vi "FeedbackDecode_20200902.vi"() -> ()   [LabVIEW 2016] (continued)
  out "prevWAVChart":dbl[](graph)=[0.01885986328125, 0.02471923828125, 0.026458740234375, 0.019622802734375, 0.015625, 0.016571044921875, 0.017852783203125, 0.016937255859375, 0.02349853515625, 0.0262451171875, 0.021697998046875, 0.01995849609375, 0.013427734375, 0.008819580078125, 0.013916015625, 0.016693115234375, 0.0172119140625, 0.023468017578125, 0.0235595703125, 0.018890380859375, 0.022369384765625, 0.022003173828125, 0.019378662109375, 0.017578125, 0.0115966796875, 0.011688232421875, 0.011016845703125, 0.007659912109375, 0.012359619140625, 0.015167236328125, 0.010162353515625, 0.00787353515625, 0.010009765625, 0.01434326171875, 0.018524169921875, 0.019012451171875, 0.019317626953125, 0.019500732421875, 0.021514892578125, 0.021514892578125, 0.0233154296875, 0.02276611328125, 0.0174560546875, 0.018585205078125, 0.019439697265625, 0.01959228515625, 0.0185546875, 0.015594482421875, 0.01593017578125, 0.0162353515625, 0.013427734375, 0.01519775390625, 0.005340576171875, 0.008026123046875, 0.00811767578125, 0.004669189453125, 0.008148193359375, 0.00384521484375, 0.007598876953125, 0.007354736328125, 0.009735107421875, 0.01580810546875, 0.01385498046875, 0.014923095703125, 0.00830078125, 0.005096435546875, 0.008941650390625, 0.01416015625, 0.01220703125, 0.0140380859375, 0.01275634765625, 0.006439208984375, 0.007049560546875, 0.006134033203125, -0.000457763671875, 0.003326416015625, 0.0081787109375, 0.009124755859375, 0.013458251953125, 0.014007568359375, 0.014312744140625, 0.006011962890625, 0.00238037109375, 0.010284423828125, 0.011962890625, 0.009857177734375, 0.00909423828125, 0.016448974609375, 0.01885986328125, 0.01190185546875, 0.010955810546875, 0.01019287109375, 0.00152587890625, 0.00762939453125, 0.008270263671875, 0.00604248046875, 0.010589599609375, 0.0037841796875, 0.0050048828125, 0.007080078125, 0.004669189453125, 0.0064697265625, 0.01068115234375, 0.009521484375, 0.002532958984375, -0.000518798828125, 0.005035400390625, 0.0042724609375, 0.00164794921875, 0.0001220703125, -0.002716064453125, -0.00164794921875, -0.007232666015625, -0.01153564453125, -0.005889892578125, -0.00341796875, -0.008514404296875, -0.007415771484375, -0.00726318359375, -0.007781982421875, -0.009918212890625, -0.010772705078125, -0.00628662109375, -0.001373291015625, -0.0008544921875, -0.003997802734375, 0.003021240234375, 0.003082275390625, 0.000640869140625, 0.00250244140625, 0.002960205078125, 0.00115966796875, 0.000579833984375, -0.002166748046875, -0.00115966796875, -0.006591796875, -0.0128173828125, -0.013275146484375, -0.0157470703125, -0.016204833984375, -0.013885498046875, -0.01531982421875, -0.00897216796875, -0.00762939453125, -0.00738525390625, -0.00311279296875, -0.002166748046875, 0.000244140625, -0.003509521484375, -0.003662109375, 0.001220703125, 0.001251220703125, 0.0001220703125, -0.003692626953125, -0.003997802734375, -0.004364013671875, -9.1552734375e-05, 0.00341796875, 0.000457763671875, -0.000274658203125, -0.0006103515625, 0.00543212890625, 0.001312255859375, 0.003662109375, 0.009765625, 0.004852294921875, 0.003997802734375, 0.00189208984375, -0.000213623046875, -0.006500244140625, -0.006744384765625, -0.0120849609375, -0.012359619140625, -0.003631591796875, -0.005645751953125, -0.0028076171875, 0.00286865234375, -0.00311279296875, -0.005279541015625, 0.001922607421875, -0.003753662109375, -0.000335693359375, -0.00299072265625, 0.001556396484375, 0.00299072265625, 0.006317138671875, 0.006622314453125, -0.003692626953125, -0.007110595703125, 0.001190185546875, -0.002288818359375, 0.00030517578125, 0.007720947265625, 0.003692626953125, 0.006011962890625, 0.007904052734375, 0.0115966796875, 0.01513671875, 0.00421142578125, 0.00299072265625, 0.002532958984375, 0.0009765625, 0.0018310546875, 0.001556396484375, 0.00640869140625, 0.008148193359375, 0.011962890625, 0.01416015625, 0.01055908203125, 0.0126953125, 0.006500244140625, 0.00958251953125, 0.009613037109375, 0.00921630859375, 0.007049560546875, 0.00927734375, 0.011871337890625, 0.015655517578125, 0.0146484375, 0.011627197265625, 0.0162353515625, 0.007965087890625, 0.00146484375, 0.004425048828125, 0.007415771484375, 0.007598876953125, 0.011810302734375, 0.01324462890625, 0.016357421875, 0.0126953125, 0.012451171875, 0.01763916015625, 0.0196533203125, 0.019775390625, 0.021453857421875, 0.025848388671875, 0.023468017578125, 0.01934814453125, 0.019073486328125, 0.020355224609375, 0.021270751953125, 0.024139404296875, 0.02545166015625, 0.0255126953125, 0.027862548828125, 0.027435302734375, 0.030487060546875, 0.029052734375, 0.032196044921875, 0.030120849609375, 0.035552978515625, 0.026611328125, 0.025787353515625, 0.030303955078125, 0.021270751953125, 0.027099609375, 0.032379150390625, 0.03143310546875, 0.02508544921875, 0.03118896484375, 0.029510498046875, 0.0311279296875, 0.03460693359375, 0.0340576171875, 0.027435302734375, 0.03076171875, 0.031707763671875, 0.029815673828125, 0.0341796875, 0.039337158203125, 0.0396728515625, 0.039459228515625, 0.031463623046875, 0.025482177734375, 0.03057861328125, 0.031707763671875, 0.03253173828125, 0.035308837890625, 0.0355224609375, 0.035369873046875, 0.02996826171875, 0.0267333984375, 0.025665283203125, 0.024688720703125, 0.029754638671875, 0.023681640625, 0.02490234375, 0.026458740234375, 0.025726318359375, 0.03436279296875, 0.028411865234375, 0.0225830078125, 0.02349853515625, 0.021270751953125, 0.02691650390625, 0.02520751953125, 0.023101806640625, 0.020782470703125, 0.0198974609375, 0.024200439453125, 0.021148681640625, 0.023406982421875, 0.028289794921875, 0.02862548828125, 0.03240966796875, 0.025634765625, 0.030120849609375, 0.029998779296875, 0.02752685546875, 0.033660888671875, 0.028167724609375, 0.032073974609375, 0.033233642578125, 0.02862548828125, 0.029876708984375, 0.02667236328125, 0.02392578125, 0.02764892578125, 0.026275634765625, 0.023468017578125, 0.031158447265625, 0.0306396484375, 0.022125244140625, 0.022430419921875, 0.025054931640625, 0.02337646484375, 0.025299072265625, 0.02777099609375, 0.03326416015625, 0.02777099609375, 0.025390625, 0.028778076171875, 0.02239990234375, 0.01837158203125, 0.021148681640625, 0.021514892578125, 0.018218994140625, 0.01593017578125, 0.017547607421875, 0.018524169921875, 0.01739501953125, 0.01922607421875, 0.016632080078125, 0.010772705078125, 0.013519287109375, 0.011383056640625, 0.013671875, 0.017242431640625, 0.021636962890625, 0.01922607421875, 0.01593017578125, 0.016571044921875, 0.015777587890625, 0.016693115234375, 0.011260986328125, 0.005828857421875, 0.0068359375, 0.001739501953125, 0.00518798828125, 0.006591796875, 0.00286865234375, 0.015289306640625, 0.011383056640625, 0.01031494140625, 0.00927734375, 0.009307861328125, 0.011199951171875, 0.010894775390625, 0.006927490234375, 0.0115966796875, 0.004638671875, 0.004425048828125, 0.003631591796875, 0.007659912109375, 0.0086669921875, 0.00616455078125, 0.003509521484375, -0.000518798828125, 0.0001220703125, -0.001708984375, -0.0015869140625, 0.002349853515625, 0.0089111328125, 0.007171630859375, 0.0072021484375, 0.004791259765625, 0.00341796875, 0.001068115234375, 0.00341796875, 0.00445556640625, 0.008056640625, 0.009246826171875, 0.011077880859375, 0.006195068359375, 0.005340576171875, 0.00244140625, 0.006561279296875, 0.016021728515625, 0.011322021484375, 0.0079345703125, 0.006622314453125, 0.01080322265625, 0.009796142578125, 0.0028076171875, 0.00439453125, 0.00048828125, 0.0052490234375, 0.0025634765625, 0.00396728515625, 0.0057373046875, 0.00860595703125, 0.00701904296875, 0.0020751953125, -0.00189208984375, -0.001861572265625, 0.00091552734375, -0.00762939453125, -0.0074462890625, -0.0054931640625, 0.0010986328125, 0.00421142578125, 0.001800537109375, 0.007232666015625, -0.001190185546875, 9.1552734375e-05, -0.0078125, -0.010833740234375, -0.0068359375, -0.0054931640625, -0.004791259765625, -0.011016845703125, -0.009765625, -0.007720947265625, -0.00384521484375, -0.011260986328125, -0.00848388671875, -0.000152587890625, -0.00030517578125, -0.00177001953125, -0.0052490234375, -0.00994873046875, -0.001617431640625, -0.00567626953125, -0.008209228515625, -0.004638671875, -0.0057373046875, -0.0067138671875, -0.01080322265625, -0.008544921875, -0.0120849609375, -0.009857177734375, -0.01409912109375, -0.0184326171875, -0.022003173828125, -0.023101806640625, -0.02197265625, -0.021942138671875, -0.018035888671875, -0.016632080078125, -0.025726318359375, -0.032623291015625, -0.02557373046875, -0.03179931640625, -0.020660400390625, -0.017578125, -0.01641845703125, -0.017852783203125, -0.02423095703125, -0.030609130859375, -0.03009033203125, -0.027862548828125, -0.031646728515625, -0.03076171875, -0.0225830078125, -0.015472412109375, -0.018341064453125, -0.02520751953125, -0.032958984375, -0.034759521484375, -0.034637451171875, -0.033233642578125, -0.031768798828125, -0.025238037109375, -0.02752685546875, -0.03057861328125, -0.0286865234375, -0.03204345703125, -0.02850341796875, -0.020965576171875, -0.022735595703125, -0.02435302734375, -0.024383544921875, -0.02496337890625, -0.01910400390625, -0.0230712890625, -0.0225830078125, -0.02435302734375, -0.027984619140625, -0.027740478515625, -0.026153564453125, -0.03021240234375, -0.030792236328125, -0.0277099609375, -0.0250244140625, -0.02239990234375, -0.025146484375, -0.029571533203125, -0.022491455078125, -0.02587890625, -0.02081298828125, -0.024688720703125, -0.026885986328125, -0.026214599609375, -0.025482177734375, -0.027374267578125, -0.03387451171875, -0.03570556640625, -0.0379638671875, -0.03662109375, -0.034637451171875, -0.03826904296875, -0.0408935546875, -0.037384033203125, -0.038177490234375, -0.039337158203125, -0.03564453125, -0.02972412109375, -0.02410888671875, -0.01873779296875, -0.02288818359375, -0.02679443359375, -0.03839111328125, -0.0316162109375, -0.029449462890625, -0.02972412109375, -0.03564453125, -0.034332275390625, -0.038665771484375, -0.044525146484375, -0.040374755859375, -0.039031982421875, -0.03741455078125, -0.039703369140625, -0.0386962890625, -0.036834716796875, -0.03521728515625, -0.033905029296875, -0.02984619140625, -0.035430908203125, -0.032440185546875, -0.029022216796875, -0.024688720703125, -0.024139404296875, -0.027099609375, -0.027313232421875, -0.02496337890625, -0.02203369140625, -0.0244140625, -0.021240234375, -0.02392578125, -0.020782470703125, -0.01873779296875, -0.0208740234375, -0.0208740234375, -0.022491455078125, -0.01806640625, -0.0216064453125, -0.017181396484375, -0.01397705078125, -0.01556396484375, -0.009979248046875, -0.016693115234375, -0.01068115234375, -0.016754150390625, -0.01959228515625, -0.016143798828125, -0.02447509765625, -0.029266357421875, -0.026947021484375, -0.02496337890625, -0.0345458984375, -0.027618408203125, -0.0318603515625, -0.028656005859375, -0.02685546875, -0.025634765625, -0.02392578125, -0.026031494140625, -0.014617919921875, -0.018585205078125, -0.021697998046875, -0.019317626953125, -0.02044677734375, -0.0184326171875, -0.018951416015625, -0.022125244140625, -0.019073486328125, -0.02203369140625, -0.0224609375, -0.02166748046875, -0.019073486328125, -0.015411376953125, -0.016448974609375, -0.023834228515625, -0.021728515625, -0.016387939453125, -0.009490966796875, -0.012542724609375, -0.0169677734375, -0.017822265625, -0.02105712890625, -0.017913818359375, -0.016815185546875, -0.01983642578125, -0.0179443359375, -0.0123291015625, -0.01129150390625, -0.01324462890625, -0.015869140625, -0.01385498046875, -0.016387939453125, -0.015655517578125, -0.0181884765625, -0.017578125, -0.013092041015625, -0.008331298828125, -0.007781982421875, -0.00439453125, -0.007080078125, -0.010223388671875, -0.01239013671875, -0.014923095703125, -0.01080322265625, -0.001983642578125, -0.0074462890625, -0.017791748046875, -0.023040771484375, -0.02978515625, -0.0267333984375, -0.0224609375, -0.017120361328125, -0.024871826171875, -0.01788330078125, -0.012298583984375, -0.011566162109375, -0.00726318359375, -0.00457763671875, -0.00299072265625, 0.00146484375, -0.0037841796875, -0.008819580078125, -0.0076904296875, -0.006256103515625, 0.001373291015625, -0.001708984375, -0.00335693359375, 0.001953125, 0.005859375, 0.00396728515625, 0.007110595703125, 0.011993408203125, 0.005828857421875, 0.00677490234375, 0.000244140625, 0.008575439453125, 0.0098876953125, 0.003875732421875, 0.0067138671875, 0.000946044921875, 0.00274658203125, 0.001800537109375, 0.00506591796875, 0.006072998046875, -0.006103515625, -0.00909423828125, -0.003936767578125, -0.001861572265625, -0.002777099609375, 0.001495361328125, 0.0006103515625, -0.003265380859375, -0.0003662109375, 0.00128173828125, 0.0010986328125, 0.002655029296875, -0.005615234375, -0.01275634765625, -0.00775146484375, -0.004913330078125, -0.004119873046875, -0.00506591796875, -9.1552734375e-05, 0.003204345703125, -0.002410888671875, -0.001800537109375, 0.001312255859375, 0.003173828125, -0.002899169921875, -0.004608154296875, 0.002593994140625, -0.002685546875, -0.00762939453125, -0.0028076171875, -0.006805419921875, -0.0146484375, -0.009979248046875, -0.00177001953125, 0.00286865234375, -0.0091552734375, -0.01495361328125, -0.01080322265625, -0.009368896484375, 0.0023193359375, -0.0010986328125, -0.001678466796875, -0.00177001953125, -0.006134033203125, -0.004730224609375, -0.00921630859375, -0.00909423828125, -0.0108642578125, -0.017181396484375, -0.015289306640625, -0.01458740234375, -0.013336181640625, -0.0057373046875, -0.004852294921875, -0.005645751953125, -0.0050048828125, -0.006500244140625, -0.00927734375, -0.012908935546875, -0.014404296875, -0.0155029296875, -0.0115966796875, -0.009796142578125, -0.01202392578125, -0.018157958984375, -0.021240234375, -0.015533447265625, -0.01629638671875, -0.01318359375, -0.015594482421875, -0.020721435546875, -0.017974853515625, -0.02056884765625, -0.02264404296875, -0.01654052734375, -0.01702880859375, -0.0146484375, -0.013275146484375, -0.023040771484375, -0.015960693359375, -0.013092041015625, -0.011077880859375, -0.009063720703125, -0.01727294921875, -0.018035888671875, -0.01580810546875, -0.011932373046875, -0.01287841796875, -0.003692626953125, -0.015167236328125, -0.014068603515625, -0.01666259765625, -0.0211181640625, -0.01812744140625, -0.013336181640625, -0.01519775390625, -0.0093994140625, -0.012847900390625, -0.0208740234375, -0.01300048828125, -0.006988525390625, -0.006072998046875, -0.011199951171875, -0.01263427734375, -0.01263427734375, -0.015625, -0.01055908203125, -0.00372314453125, -0.001312255859375, 0.001861572265625, -6.103515625e-05, -0.00311279296875, -0.001251220703125, -0.006500244140625, -0.00665283203125, 0.000823974609375, 0.001190185546875, 0.004486083984375, -0.004638671875, -0.00250244140625, -0.000518798828125, 0.001739501953125, 0.010955810546875, 0.00384521484375, -0.002349853515625, -0.00128173828125, -0.002227783203125, -0.005157470703125, -0.003204345703125, -0.00482177734375, -0.006072998046875, -0.001312255859375, -0.00018310546875, 0.0001220703125, -0.000274658203125, 0.003753662109375, 0.0103759765625, 0.009063720703125, 0.01324462890625, 0.019989013671875, 0.01324462890625, 0.015350341796875, 0.017791748046875, 0.019744873046875, 0.0157470703125, 0.007049560546875, 0.01263427734375, 0.0111083984375, 0.009002685546875, 0.01141357421875, 0.016632080078125, 0.012847900390625, 0.007568359375, 0.0042724609375, -0.00372314453125, -0.011383056640625, 0.00128173828125, 0.014312744140625, 0.016082763671875, 0.021697998046875, 0.020172119140625, 0.021575927734375, 0.02032470703125, 0.02215576171875, 0.02471923828125, 0.0302734375, 0.02752685546875, 0.02667236328125, 0.026580810546875, 0.0250244140625, 0.027557373046875, 0.020172119140625, 0.0247802734375, 0.02978515625, 0.030120849609375, 0.03131103515625, 0.031524658203125, 0.032257080078125, 0.0286865234375, 0.03033447265625, 0.0279541015625, 0.03582763671875, 0.036285400390625, 0.03515625, 0.028656005859375, 0.0311279296875, 0.033599853515625, 0.03582763671875, 0.028839111328125, 0.02947998046875, 0.0306396484375, 0.025146484375, 0.020843505859375, 0.027679443359375, 0.028045654296875, 0.02532958984375, 0.024017333984375, 0.02410888671875, 0.032073974609375, 0.018951416015625, 0.02801513671875, 0.0318603515625, 0.02587890625, 0.02825927734375, 0.025421142578125, 0.033203125, 0.03515625, 0.0362548828125, 0.030975341796875, 0.034332275390625, 0.02392578125, 0.027191162109375, 0.03472900390625, 0.03515625, 0.02813720703125, 0.0291748046875, 0.028717041015625, 0.027099609375, 0.02874755859375, 0.02203369140625, 0.019805908203125, 0.0179443359375, 0.0289306640625, 0.023773193359375, 0.017059326171875, 0.020904541015625, 0.0262451171875, 0.022979736328125, 0.021453857421875, 0.024017333984375, 0.02056884765625, 0.022430419921875, 0.02081298828125, 0.021759033203125, 0.026611328125, 0.033660888671875, 0.027374267578125, 0.02435302734375, 0.0185546875, 0.018096923828125, 0.023223876953125, 0.01654052734375, 0.015899658203125, 0.009490966796875, 0.00897216796875, 0.00933837890625, 0.013763427734375, 0.01470947265625, 0.021392822265625, 0.0238037109375, 0.022979736328125, 0.025665283203125, 0.0169677734375, 0.0174560546875, 0.015472412109375, 0.012786865234375, 0.011688232421875, 0.0103759765625, 0.00640869140625, 0.0113525390625, 0.0142822265625, 0.012603759765625, 0.0142822265625, 0.016815185546875, 0.020782470703125, 0.012237548828125, 0.008392333984375, 0.017578125, 0.019775390625, 0.026336669921875, 0.02557373046875, 0.019317626953125, 0.015380859375, 0.0196533203125, 0.01812744140625, 0.020050048828125, 0.015045166015625, 0.01416015625, 0.01129150390625, 0.00885009765625, 0.00799560546875, 0.01055908203125, 0.0107421875, 0.0164794921875, 0.0133056640625, 0.0064697265625, 0.0089111328125, 0.0069580078125, 0.0064697265625, 0.001220703125, -0.003082275390625, -0.0028076171875, -9.1552734375e-05, 0.00201416015625, -0.000946044921875, -0.001495361328125, 0.000579833984375, 0.003265380859375, 0.00390625, 0.005889892578125, 0.002685546875, -0.000732421875, 0.004058837890625, 0.0023193359375, 0.008544921875, 0.00250244140625, -0.000885009765625, -0.00244140625, -0.004608154296875, -0.002288818359375, -0.0050048828125, -0.000885009765625, -0.0013427734375, 0.001800537109375, 0.001678466796875, -0.005279541015625, 0.00506591796875, 0.002899169921875, 0.003662109375, 0.0087890625, 0.011474609375, 0.01422119140625, 0.01055908203125, 0.011444091796875, 0.012359619140625, 0.001190185546875, 0.0054931640625, 0.007598876953125, 0.01025390625, 0.01300048828125, 0.008575439453125, 0.007659912109375, 0.00897216796875, 0.014892578125, 0.01226806640625, 0.014434814453125, 0.022003173828125, 0.02056884765625, 0.022705078125, 0.02532958984375, 0.02154541015625, 0.02130126953125, 0.01788330078125, 0.016845703125, 0.018524169921875, 0.015167236328125, 0.01947021484375, 0.017578125, 0.01470947265625, 0.015533447265625, 0.015594482421875, 0.00836181640625, 0.0164794921875, 0.017608642578125, 0.012481689453125, 0.01287841796875, 0.01123046875, 0.010986328125, 0.01324462890625, 0.015655517578125, 0.01287841796875, 0.0107421875, 0.012908935546875, 0.00885009765625, 0.00201416015625, 0.008026123046875, 0.00994873046875, 0.011444091796875, 0.010894775390625, 0.01385498046875, 0.0174560546875, 0.014495849609375, 0.009246826171875, 0.00982666015625, 0.010406494140625, 0.015411376953125, 0.01507568359375, 0.0067138671875, 0.009521484375, 0.011322021484375, 0.00811767578125, -0.002410888671875, 0.00299072265625, -0.004852294921875, 0.0032958984375, 0.0032958984375, 6.103515625e-05, 0.00152587890625, 0.003082275390625, 0.011627197265625, 0.013458251953125, 0.01239013671875, 0.015777587890625, 0.023406982421875, 0.027923583984375, 0.024139404296875, 0.020721435546875, 0.022308349609375, 0.026519775390625, 0.019256591796875, 0.013214111328125, 0.0146484375, 0.015777587890625, 0.02001953125, 0.0150146484375, 0.01055908203125, 0.00897216796875, 0.00823974609375, 0.0013427734375, 0.005615234375, -0.00225830078125, -0.008087158203125, 0.005950927734375, 0.00762939453125, 0.003326416015625, 0.009002685546875, 0.006744384765625, 0.0101318359375, 0.00732421875, 0.004425048828125, 0.01068115234375, 0.001251220703125, 0.008758544921875, 0.018218994140625, 0.013885498046875, 0.014617919921875, 0.011383056640625, 0.01373291015625, 0.0115966796875, 0.00567626953125, 0.002716064453125, -0.000823974609375, 0.0025634765625, 0.0028076171875, 0.002044677734375, -0.000335693359375, 0.0029296875, 0.002655029296875, 0.002349853515625, 0.001678466796875, 0.00433349609375, 0.011871337890625, 0.006744384765625, 0.001129150390625, 0.000640869140625, -0.00042724609375, -0.007781982421875, -0.00433349609375, -0.002166748046875, 0.00189208984375, 0.000823974609375, -0.001922607421875, -0.000152587890625, -0.001007080078125, -0.005035400390625, -0.006439208984375, -0.00799560546875, -0.0150146484375, -0.017822265625, -0.02020263671875, -0.012542724609375, -0.01116943359375, -0.012298583984375, -0.017974853515625, -0.011810302734375, -0.009674072265625, -0.01446533203125, -0.0096435546875, -0.017852783203125, -0.0228271484375, -0.024505615234375, -0.022064208984375, -0.01568603515625, -0.01495361328125, -0.017242431640625, -0.014862060546875, -0.011871337890625, -0.009979248046875, -0.007965087890625, -0.007598876953125, -0.00628662109375, -0.009613037109375, -0.00982666015625, -0.0140380859375, -0.013275146484375, -0.016510009765625, -0.02313232421875, -0.019744873046875, -0.02117919921875, -0.024261474609375, -0.023406982421875, -0.025634765625, -0.026123046875, -0.029937744140625, -0.0272216796875, -0.025054931640625, -0.0198974609375, -0.020263671875, -0.022705078125, -0.0177001953125, -0.018585205078125, -0.020751953125, -0.01678466796875, -0.017181396484375, -0.016937255859375, -0.01995849609375, -0.014312744140625, -0.015350341796875, -0.016815185546875, -0.014129638671875, -0.02496337890625, -0.019317626953125, -0.023193359375, -0.017059326171875, -0.015533447265625, -0.020843505859375, -0.01788330078125, -0.021575927734375, -0.016876220703125, -0.0162353515625, -0.01556396484375, -0.02313232421875, -0.017822265625, -0.011871337890625, -0.0125732421875, -0.01348876953125, -0.014312744140625, -0.00909423828125, -0.009063720703125, -0.010345458984375, -0.00726318359375, -0.01397705078125, -0.009490966796875, -0.00982666015625, -0.007598876953125, -0.00421142578125, -0.00067138671875, 0.001953125, 0.001556396484375, 0.001220703125, -0.009185791015625, -0.013336181640625, -0.01556396484375, -0.01116943359375, -0.0096435546875, -0.010162353515625, -0.011749267578125, -0.012359619140625, -0.009124755859375, -0.009857177734375, -0.011474609375, -0.007568359375, -0.0068359375, -0.0062255859375, -0.00482177734375, -0.010467529296875, -0.0078125, -0.00750732421875, -0.01434326171875, -0.01361083984375, -0.0181884765625, -0.020782470703125, -0.007568359375, -0.006988525390625, -0.006622314453125, -0.001861572265625, -0.00128173828125, -0.0115966796875, -0.005401611328125, -0.004974365234375, -0.0084228515625, -0.011383056640625, -0.0118408203125, -0.008148193359375, -0.006256103515625, -0.001861572265625, 0.004302978515625, 0.004913330078125, 0.006195068359375, 0.00897216796875, 0.003753662109375, 0.00360107421875, -0.00201416015625, -0.001190185546875, -0.0030517578125, -0.0067138671875, -0.00469970703125, -0.005828857421875, -0.005645751953125, 0.001708984375, 0.002960205078125, 0.005767822265625, 0.001983642578125, 0.00048828125, -0.00103759765625, -0.001556396484375, 0.0, 0.007659912109375, 0.01202392578125, 0.010986328125, 0.0059814453125, 0.007354736328125, 0.01275634765625, 0.010009765625, 0.008880615234375, 0.008544921875, 0.007354736328125, 0.001800537109375, 0.00115966796875, -0.002410888671875, 0.009063720703125, 0.01190185546875, 0.012908935546875, 0.010650634765625, 0.004974365234375, 0.01251220703125, 0.012603759765625, 0.007110595703125, 0.00860595703125, 0.017303466796875, 0.01348876953125, 0.01556396484375, 0.0159912109375, 0.0147705078125, 0.01861572265625, 0.014068603515625, 0.0167236328125, 0.015533447265625, 0.0198974609375, 0.019866943359375, 0.015350341796875, 0.0079345703125, 0.0091552734375, 0.00921630859375, 0.011077880859375, 0.00738525390625, 0.008544921875, 0.01690673828125, 0.01513671875, 0.010009765625, 0.0107421875, 0.009674072265625, 0.0142822265625, 0.015899658203125, 0.012359619140625, 0.0203857421875, 0.02166748046875, 0.02032470703125, 0.02069091796875, 0.018280029296875, 0.010772705078125, 0.0057373046875, 0.013519287109375, 0.017242431640625, 0.011383056640625, 0.0142822265625, 0.013824462890625, 0.011962890625, 0.010284423828125, 0.0089111328125, 0.011993408203125, 0.0103759765625, -3.0517578125e-05, -0.00640869140625, -0.00506591796875, -0.00701904296875, -0.003143310546875, 0.0037841796875, 0.008209228515625, 0.00518798828125, 0.00506591796875, 0.006591796875, 0.00701904296875, 0.00567626953125, 0.011383056640625, 0.00543212890625, 0.001556396484375, 0.009185791015625, 0.00628662109375, 0.009521484375, 0.01324462890625, 0.0198974609375, 0.01837158203125, 0.017669677734375, 0.0103759765625, 0.013214111328125, 0.015594482421875, 0.014495849609375, 0.013092041015625, 0.010711669921875, 0.006195068359375, 0.0054931640625, 0.012969970703125, 0.01123046875, 0.017974853515625, 0.015106201171875, 0.011505126953125, 0.009307861328125, 0.024322509765625, 0.023284912109375, 0.01983642578125, 0.025726318359375, 0.030059814453125, 0.0242919921875, 0.02655029296875, 0.03326416015625, 0.023712158203125, 0.02374267578125, 0.022552490234375, 0.0157470703125, 0.020782470703125, 0.022064208984375, 0.022430419921875, 0.0272216796875, 0.02301025390625, 0.019744873046875, 0.018768310546875, 0.0240478515625, 0.029876708984375, 0.032196044921875, 0.030975341796875, 0.026458740234375, 0.025421142578125, 0.023529052734375, 0.024505615234375, 0.021697998046875, 0.018768310546875, 0.0145263671875, 0.01544189453125, 0.0244140625, 0.0198974609375, 0.017578125, 0.021148681640625, 0.01885986328125, 0.0191650390625, 0.018890380859375, 0.02740478515625, 0.018646240234375, 0.02069091796875, 0.025787353515625, 0.02423095703125, 0.0245361328125, 0.022796630859375, 0.01898193359375, 0.01727294921875, 0.021514892578125, 0.014739990234375, 0.01812744140625, 0.023651123046875, 0.020263671875, 0.01995849609375, 0.01971435546875, 0.021331787109375, 0.013336181640625, 0.01605224609375, 0.020111083984375, 0.0228271484375, 0.01959228515625, 0.0181884765625, 0.02130126953125, 0.00885009765625, 0.0120849609375, 0.012786865234375, 0.01593017578125, 0.021728515625, 0.021636962890625, 0.02227783203125, 0.017791748046875, 0.01885986328125, 0.025177001953125, 0.027557373046875, 0.019287109375, 0.01025390625, 0.01348876953125, 0.014129638671875, 0.02435302734375, 0.026336669921875, 0.02685546875, 0.0263671875, 0.029052734375, 0.03204345703125, 0.026580810546875, 0.033050537109375, 0.03021240234375, 0.02557373046875, 0.02392578125, 0.027801513671875, 0.0362548828125, 0.036041259765625, 0.03271484375, 0.03167724609375, 0.0325927734375, 0.038818359375, 0.036163330078125, 0.037017822265625, 0.030364990234375, 0.02996826171875, 0.029754638671875, 0.02813720703125, 0.021087646484375, 0.02264404296875, 0.020782470703125, 0.02197265625, 0.026580810546875, 0.020111083984375, 0.023834228515625, 0.02264404296875, 0.018157958984375, 0.026123046875, 0.027130126953125, 0.027618408203125, 0.031829833984375, 0.030487060546875, 0.027587890625, 0.025115966796875, 0.02667236328125, 0.0299072265625, 0.030426025390625, 0.0299072265625, 0.033599853515625, 0.035491943359375, 0.0390625, 0.035369873046875, 0.029266357421875, 0.022247314453125, 0.029083251953125, 0.022186279296875, 0.017181396484375, 0.02008056640625, 0.02447509765625, 0.027984619140625, 0.020782470703125, 0.0203857421875, 0.02197265625, 0.02520751953125, 0.018524169921875, 0.01922607421875, 0.02557373046875, 0.020599365234375, 0.025421142578125, 0.02606201171875, 0.026885986328125, 0.025970458984375, 0.0262451171875, 0.024200439453125, 0.0257568359375, 0.024078369140625, 0.02227783203125, 0.027923583984375, 0.0250244140625, 0.01995849609375, 0.022369384765625, 0.020538330078125, 0.021026611328125, 0.02734375, 0.0316162109375, 0.0347900390625, 0.0272216796875, 0.03057861328125, 0.034454345703125, 0.0289306640625, 0.035491943359375, 0.033538818359375, 0.023651123046875, 0.025848388671875, 0.0223388671875, 0.018646240234375, 0.01934814453125, 0.02130126953125, 0.01800537109375, 0.01824951171875, 0.01837158203125, 0.017242431640625, 0.021148681640625, 0.02520751953125, 0.02197265625, 0.021270751953125, 0.01971435546875, 0.0244140625, 0.02313232421875, 0.0244140625, 0.0272216796875, 0.0302734375, 0.023895263671875, 0.027374267578125, 0.031097412109375, 0.0198974609375, 0.0228271484375, 0.0255126953125, 0.026031494140625, 0.025299072265625, 0.030242919921875, 0.030487060546875, 0.029571533203125, 0.02880859375, 0.02398681640625, 0.029266357421875, 0.02618408203125, 0.026947021484375, 0.022216796875, 0.022247314453125, 0.022552490234375, 0.014373779296875, 0.011444091796875, 0.011444091796875, 0.012115478515625, 0.00823974609375, 0.01446533203125, 0.008636474609375, 0.00726318359375, 0.007720947265625, 0.010406494140625, 0.008758544921875, 0.00848388671875, 0.01226806640625, 0.009368896484375, 0.00732421875, -0.000823974609375, 0.00152587890625, 0.003631591796875, 0.00640869140625, 0.015655517578125, 0.0234375, 0.015960693359375, 0.010955810546875, 0.01055908203125, 0.009185791015625, 0.00994873046875, 0.016632080078125, 0.01751708984375, 0.015411376953125, 0.0157470703125, 0.0189208984375, 0.015167236328125, 0.009735107421875, 0.019439697265625, 0.024169921875, 0.02508544921875, 0.022308349609375, 0.020111083984375, 0.02056884765625, 0.018035888671875, 0.02093505859375, 0.018280029296875, 0.0152587890625, 0.0185546875, 0.01220703125, 0.01251220703125, 0.01544189453125, 0.01629638671875, 0.017120361328125, 0.01385498046875, 0.020416259765625, 0.017181396484375, 0.015960693359375, 0.01318359375, 0.009796142578125, 0.008148193359375, 0.01165771484375, 0.014892578125, 0.01531982421875, 0.013275146484375, 0.01507568359375, 0.0140380859375, 0.011993408203125, 0.0147705078125, 0.017547607421875, 0.013702392578125, 0.014678955078125, 0.014404296875, 0.0152587890625, 0.0140380859375, 0.01116943359375, 0.012176513671875, 0.009674072265625, 0.013153076171875, 0.013397216796875, 0.005462646484375, 0.011749267578125, 0.016021728515625, 0.010101318359375, 0.008819580078125, -0.000396728515625, 0.004852294921875, 0.000457763671875, 0.002838134765625, 0.0035400390625, -0.003662109375, 0.005950927734375, 0.00018310546875, 0.0047607421875, 0.0089111328125, 0.010345458984375, 0.005645751953125, 0.00897216796875, 0.009552001953125, 0.014862060546875, 0.012420654296875, 0.00762939453125, 0.009918212890625, 0.01318359375, 0.013824462890625, 0.01019287109375, 0.01519775390625, 0.018829345703125, 0.020782470703125, 0.022491455078125, 0.02142333984375, 0.01995849609375, 0.013580322265625, 0.01446533203125, 0.0179443359375, 0.012298583984375, 0.014556884765625, 0.01953125, 0.015777587890625, 0.017059326171875, 0.01171875, 0.01025390625, 0.020660400390625, 0.0185546875, 0.02239990234375, 0.026336669921875, 0.019989013671875, 0.01690673828125, 0.01507568359375, 0.0186767578125, 0.014434814453125, 0.01007080078125, 0.01788330078125, 0.016387939453125, 0.018280029296875, 0.016143798828125, 0.01678466796875, 0.012939453125, 0.014251708984375, 0.014923095703125, 0.01190185546875, 0.009674072265625, 0.014251708984375, 0.015106201171875, 0.008392333984375, 0.008544921875, 0.008514404296875, 0.011932373046875, 0.0032958984375, 0.002655029296875, 0.008544921875, 0.006622314453125, 0.012176513671875, 0.00640869140625, 0.008026123046875, 0.0126953125, 0.01043701171875, 0.003570556640625, 0.000457763671875, 0.001495361328125, 0.001190185546875, 0.0052490234375, 0.007659912109375, 0.00634765625, 0.003997802734375, 0.004150390625, 0.00885009765625, 0.00103759765625, 0.003936767578125, 0.00653076171875, 0.0006103515625, -0.000213623046875, 0.000579833984375, -0.001922607421875, 0.00189208984375, 0.002044677734375, 0.00689697265625, 0.005950927734375, 0.008514404296875, 0.010772705078125, 0.00347900390625, 0.008026123046875, 0.005218505859375, 0.005218505859375, 0.004669189453125, 0.011871337890625, 0.01348876953125, 0.015655517578125, 0.010223388671875, 0.0086669921875, 0.0128173828125, 0.0155029296875, 0.022369384765625, 0.018524169921875]
  out "SelWfs":dbl[][](graph)
  out "SelData":cluster{dbl, "RBuffSize":dbl, "SelData":dbl[]}[](graph)
  in  "MSMSSphere":dbl[][](array[numeric])=[[0.0, 0.0, 0.0, 0.15, 1.0, 1.0], [0.0, 0.0, 0.0, 0.15, 1.0, 1.0], [0.0, 0.0, 0.0, 0.15, 1.0, 1.0], [0.0, 0.0, 0.0, 0.15, 1.0, 1.0], [0.0, 0.0, 0.0, 0.15, 1.0, 1.0], [0.0, 0.0, 0.0, 0.15, 1.0, 1.0]] min=-1.0 max=1.0
  in  "MSMSMvnt":dbl[](array[numeric])=[0.0, 0.0, 0.0, 0.0, 0.0, 0.0, 0.0, 0.0, 0.0, 0.0, 0.0, 0.0] min=-1.0 max=1.0
  out "LVTiming":cluster{dbl, dbl}(graph)={0.01, 0.001}
  out "MLTiming":cluster{"MLCalcTime":dbl, "MLTotalTime":dbl}(graph)
  out "PSRef":refnum<vi>
  out "Outcome":enum16{"---", "Success", "Failure"}(ring)
  out "MLIP":string="155.100.90.185"
  out "LVIP":string="155.100.90.215"
  out "HoverPicPos":T14={"[0]"=1216, "[1]"=326, "[2]"=199, "[3]"=199}
  out "ExperimentDate":timestamp=timestamp(3516384370.2973766 s since 1904-01-01)
  out "LoopPeriod":u64=10
  out "LoopCnt":u64=9962
  out "TaskParameters":string
  out "TaskType":string="FeedbackDecode.vi"
  out "DatabaseUDL":path=path "E:/Data/PatientDatabase.udl"
  out "TrialParameters":string
  out "BaseCnt1":u64
  out "State":T16(ring)
  # "Ctrl-click on heat map will populate decode electrodes\nAlt-click on heat map will populate bad electrodes"
  # "Neural Purple"
  # "Neural Red"
  # "EMG"
  # "Thumb"
  # "Index"
  # "Middle"
  # "Ring"
  # "Thumb"
  # "Little"
  # "Index"
  # "ThumbInt"
  # "Middle"
  # "IndexInt"
  # "Ring"
  # "Ring Int"
  # "Little"
  # "Little Int"
  # "Wrist"
  # "WristPitch"
  # "PosFlex"
  # "PosInt"
  # "PosRoll"
  # "Radius"
  # "Color"
  # "Vis"
  # "WristYaw"
  # "WristRoll"
  # "G"
  # "T"
  # "Mode"
  # "S"
  # "Negative lag shifts feature variables left (earlier)"
  # "{[1,2,4];[5,3];[6,7,8]}"
  # "Select before apply training"
  # "1"
  # "2"
  # "3"
  # "4"
  # "5"
  # "6"
  # "7"
  # "8"
  # "1"
  # "2"
  # "3"
  # "4"
  # "1-2"
  # "1-3"
  # "1-4"
  # "2-3"
  # "2-4"
  # "3-4"
  # "DOF"
  # "Gain (F/E)"
  # "Thresh (F/E)"
  # "Mode"
  # "Spd"
  # "Thumb"
  # "Index"
  # "Middle"
  # "Ring"
  # "Little"
  # "ThumbInt"
  # "IndexInt"
  # "RingInt"
  # "LittleInt"
  # "WristPitch"
  # "WristYaw"
  # "WristRoll"
  # "Amp"
  # "Del"
  # "Rise"
  # "Hold"
  # "Value"
  # "Inc-"
  # "Inc+"
  # "Min Amp"
  # "Max Amp"
  # "Min Freq"
  # "Max Freq"
  # "Duration"
  # "Sensor Options:\n**************************************************\nCutaneous (*luke hand in parentheses):\n------------------------------------------------------------\nthumb_distal (*tip)          index_distal (*tip)     \nthumb_medial (*radial)   index_medial (*lateral)        \nthumb_proximal              index_proximal     \n\nmiddle_distal (*tip)          ring_distal (*tip)       \nmiddle_medial                 ring_medial         \nmiddle_proximal              ring_proximal     \n\npinky_distal (*tip)             palm_back (*back)\npinky_medial                    palm_side (*edge)\npinky_proximal                 palm_pinky (*distal)\n                                           palm_thumb (*proximal)\n\n\nProprioception (*luke hand in parentheses):\n-------------------------------------------------------------\nthumb_MCP (*pitch)         index_MCP  (*flexion)                             \nthumb_PIP                          \nthumb_DIP                                   \nthumb_ABD (*yaw)            index_ABD                                                                    \n\nmiddle_MCP (*mrp)          ring_MCP\n\npinky_MCP                        wrist_FLEX (*flexion)\npinky_ABD                         wrist_UDEV\n                                           wrist_PRO (*rotation)\n\n**************************************************"
  # "Stimulation Notes:\n\nFrequency and Amplitude scaled linearly:     Intensity*(max-min)+min\n\nReceptor Options:\n\"\" - standard linear mapping\n\"scaled\" - standard linear mapping, but scaled to match biofidelic SA1 max frequencies\n\"SA1\" - biofidelic stimulation that includes only positive dp/dt terms\n\"aSA\" - archived biofidelic stimulation that often rails at max frequency\n\"RA1\" - biofidelic stimulation that only fires on onset and on offset"
  # "Note: Pupillometry glasses must be connected prior to starting FeedbackDecode"
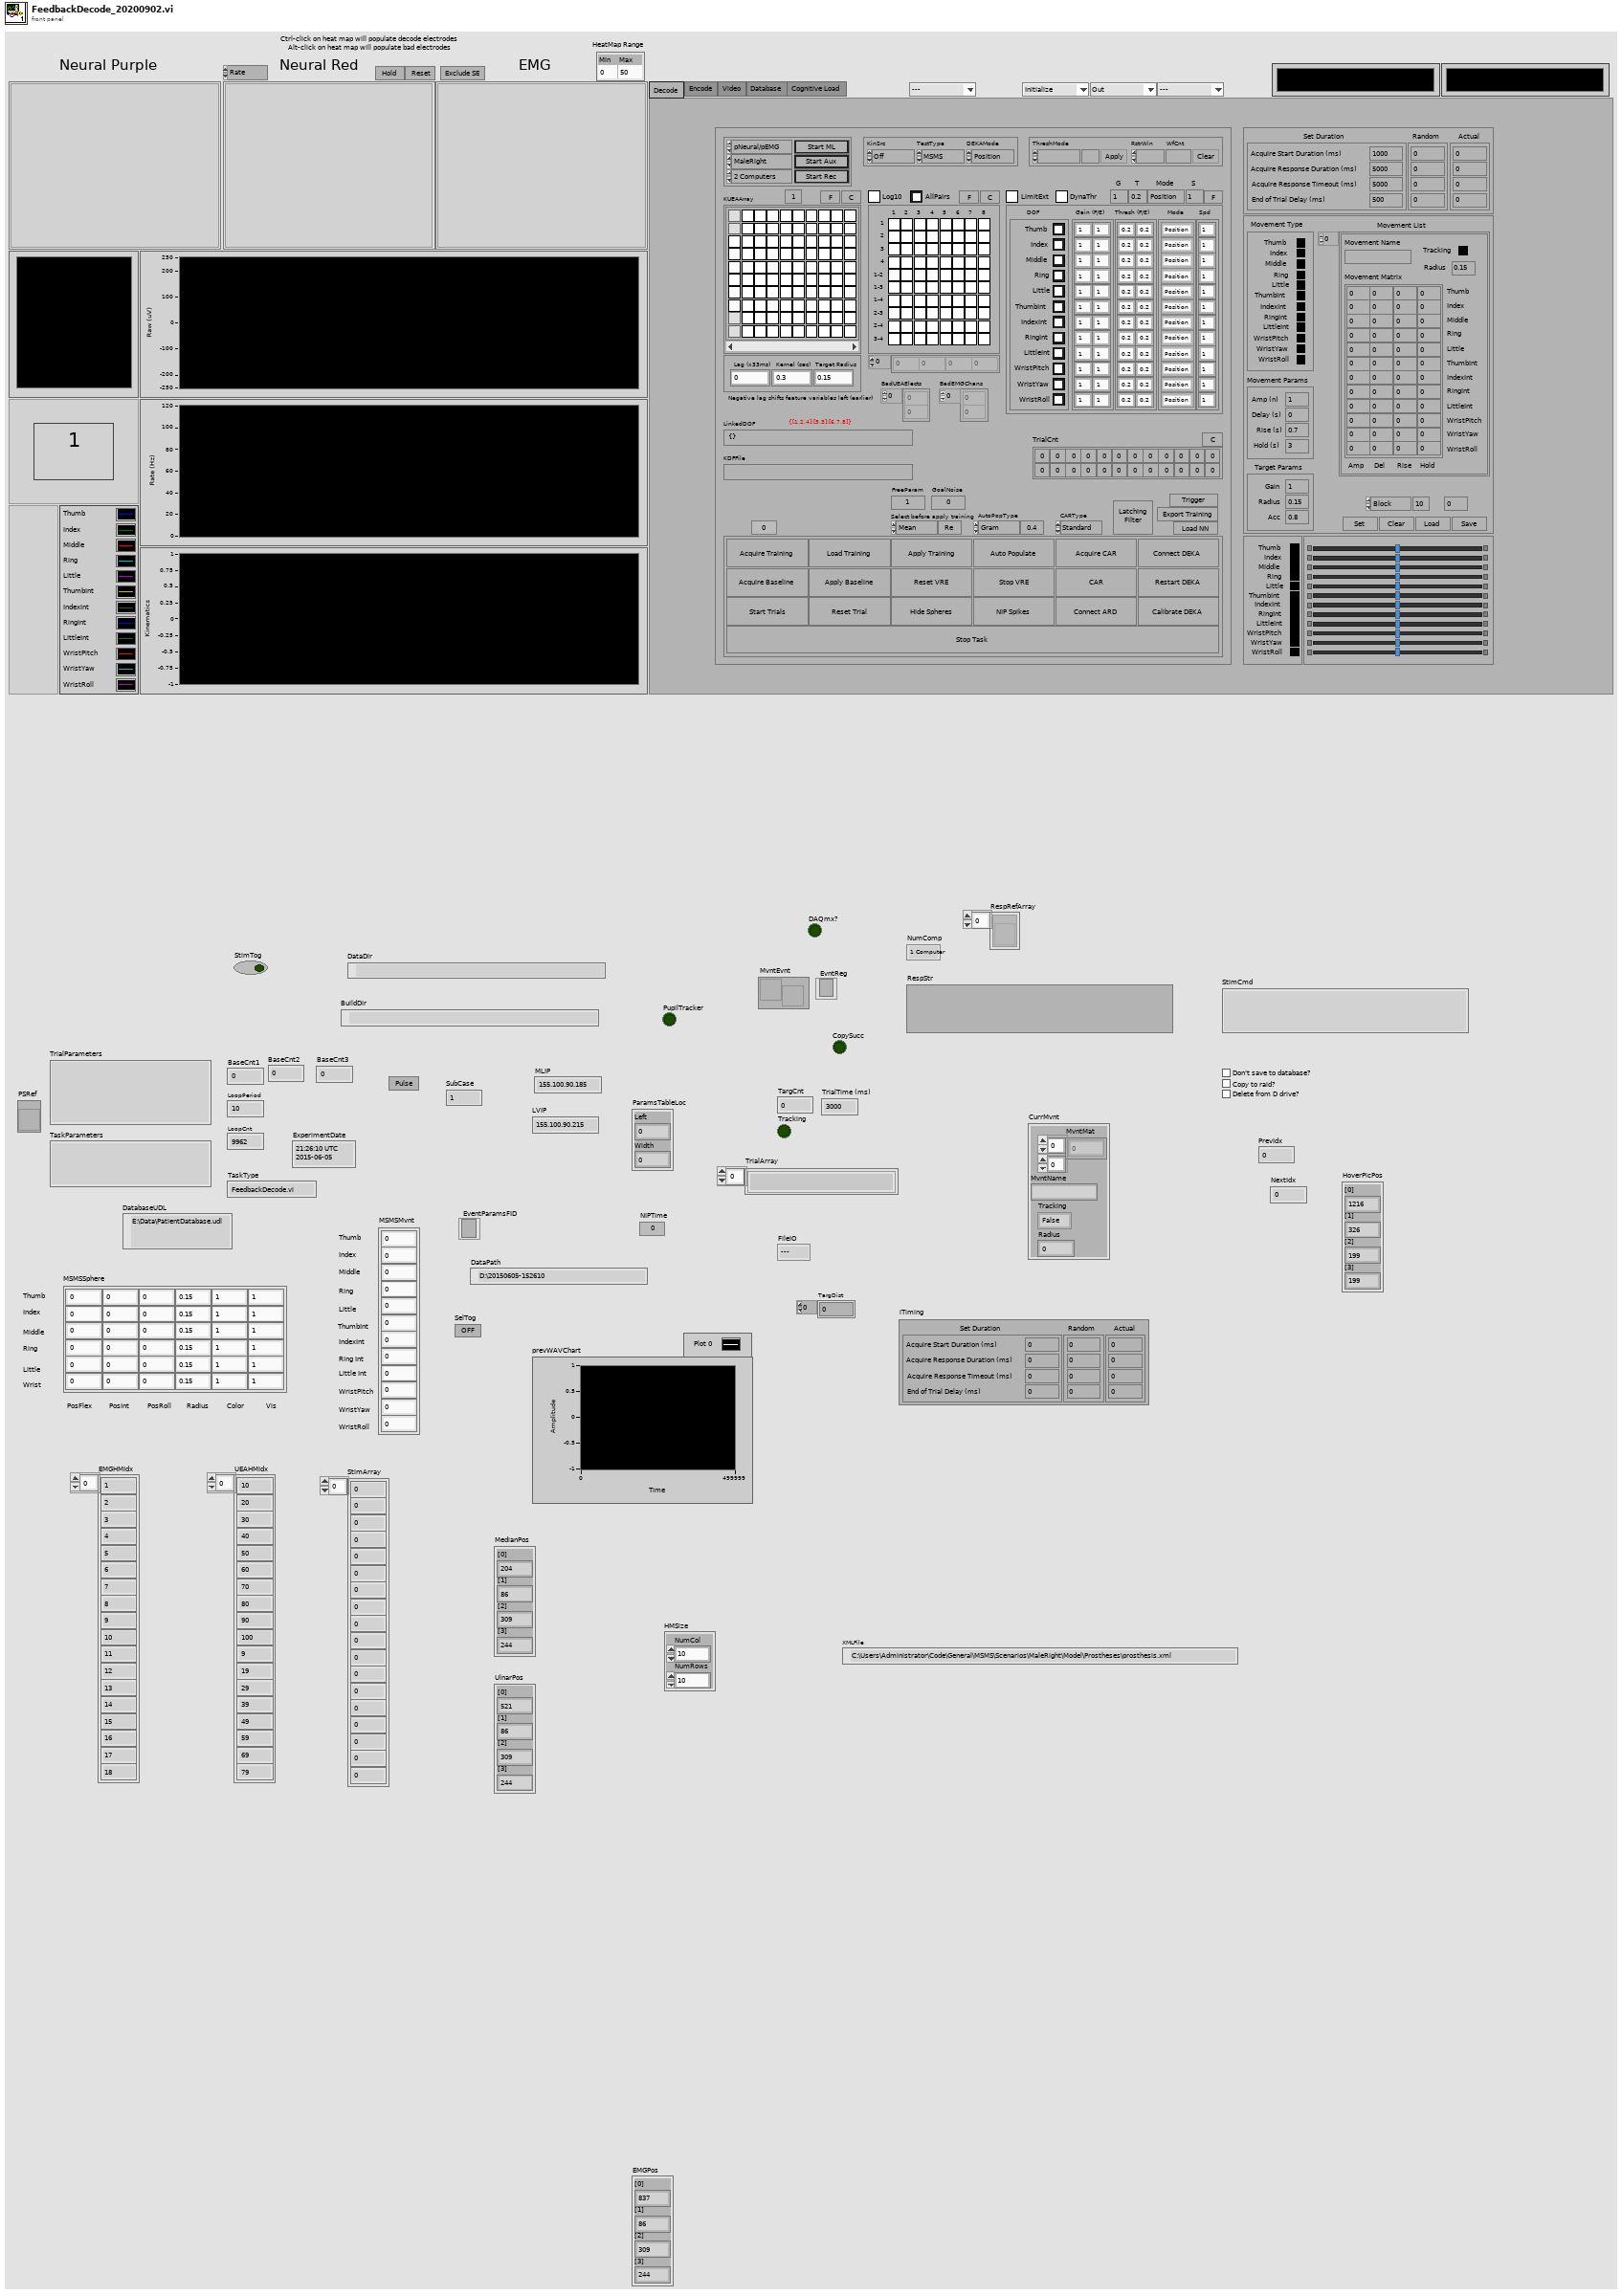
[diagram p1: front panel]
types:
  T1 = cluster{"MvntMat":dbl[][], "MvntName":string, "Tracking":enum8{"False", "True", "Mixed"}, "Radius":dbl}
  T2 = enum16{"---", "Bakeoff11", "Bakeoff21", "Bakeoff31", "Bakeoff32", "LukeEmpty", "MPLEmpty", "MPLUnknown", "MPLBasic", "MPLTarg", "LukeBasic", "FragileBlock", "mBBT"}
  T3 = cluster{"Dur":cluster{"ASD":dbl, "ARD":dbl, "ART":dbl, "ETD":dbl}, "Rnd":cluster{"ASDR":dbl, "ARDR":dbl, "ARTR":dbl, "ETDR":dbl}, "Act":cluster{"ASDA":dbl, "ARDA":dbl, "ARTA":dbl, "ETDA":dbl}}
  T4 = enum32{"Decode", "Encode", "Video", "Database", "Cognitive Load"}
  T5 = typedef "FeedbackDecode_DecodeClust.ctl" = cluster{"TrainParams":cluster{"Lag":dbl, "KernelWidth":dbl, "TargRad":dbl}, "Kinematics":cluster{"Thumb":dbl, "Index":dbl, "Middle":dbl, "Ring":dbl, "Little":dbl, "ThumbInt":dbl, "IndexInt":dbl, "RingInt":dbl, "LittleInt":dbl, "Wrist":dbl, "WristYaw":dbl, "WristRoll":dbl}, "CtrlButtons":cluster{"AcqTraining":bool, "ApplyBaseline":bool, "ApplyTraining":bool, "LoadTrainFile":bool, "CAR":bool, "NIPSpikes":bool, "AcqBaseline":bool, "Stop":bool, "ResetTrial":bool, "CalDEKA":bool, "HideSphrs":bool, "StartTrials":bool, "AutoPop":bool, "ResetVRE":bool, "StopVRE":bool, "AcqCAR":bool, "ConARD":bool, "DEKARestart":bool, "ConnDEKA":bool}, "CompID":cluster{"LV":cluster{"Name":string, "IP":string}, "ML":cluster{"Name":string, "IP":string}}, "KMvntClust":cluster{"KGain":sgl[][], "KMvnts":cluster{"Thumb":bool, "Index":bool, "Middle":bool, "Ring":bool, "Little":bool, "ThumbInt":bool, "IndexInt":bool, "RingInt":bool, "LittleInt":bool, "WristPitch":bool, "WristYaw":bool, "WristRoll":bool}, "KThresh":sgl[][], "CtrlMode":enum16{"Position", "Latching", "Leaky", "Velocity"}[], "CtrlSpd":sgl[]}, "ClearUEA":bool, "Targets":cluster{"Thumb":dbl, "Index":dbl, "Middle":dbl, "Ring":dbl, "Little":dbl, "ThumbInt":dbl, "IndexInt":dbl, "RingInt":dbl, "LittleInt":dbl, "Wrist":dbl, "WristYaw":dbl, "WristRoll":dbl}, "KUEAArray":cluster{"Boolean 1":bool, "Boolean 2":bool, "Boolean 3":bool, "Boolean 4":bool, "Boolean 5":bool, "Boolean 6":bool, "Boolean 7":bool, "Boolean 8":bool, "Boolean 9":bool, "Boolean 10":bool, "Boolean 11":bool, "Boolean 12":bool, "Boolean 13":bool, "Boolean 14":bool, "Boolean 15":bool, "Boolean 16":bool, "Boolean 17":bool, "Boolean 18":bool, "Boolean 19":bool, "Boolean 20":bool, "Boolean 21":bool, "Boolean 22":bool, "Boolean 23":bool, "Boolean 24":bool, "Boolean 25":bool, "Boolean 26":bool, "Boolean 27":bool, "Boolean 28":bool, "Boolean 29":bool, "Boolean 30":bool, "Boolean 31":bool, "Boolean 32":bool, "Boolean 33":bool, "Boolean 34":bool, "Boolean 35":bool, "Boolean 36":bool, "Boolean 37":bool, "Boolean 38":bool, "Boolean 39":bool, "Boolean 40":bool, "Boolean 41":bool, "Boolean 42":bool, "Boolean 43":bool, "Boolean 44":bool, "Boolean 45":bool, "Boolean 46":bool, "Boolean 47":bool, "Boolean 48":bool, "Boolean 49":bool, "Boolean 50":bool, "Boolean 51":bool, "Boolean 52":bool, "Boolean 53":bool, "Boolean 54":bool, "Boolean 55":bool, "Boolean 56":bool, "Boolean 57":bool, "Boolean 58":bool, "Boolean 59":bool, "Boolean 60":bool, "Boolean 61":bool, "Boolean 62":bool, "Boolean 63":bool, "Boolean 64":bool, "Boolean 65":bool, "Boolean 66":bool, "Boolean 67":bool, "Boolean 68":bool, "Boolean 69":bool, "Boolean 70":bool, "Boolean 71":bool, "Boolean 72":bool, "Boolean 73":bool, "Boolean 74":bool, "Boolean 75":bool, "Boolean 76":bool, "Boolean 77":bool, "Boolean 78":bool, "Boolean 79":bool, "Boolean 80":bool, "Boolean 81":bool, "Boolean 82":bool, "Boolean 83":bool, "Boolean 84":bool, "Boolean 85":bool, "Boolean 86":bool, "Boolean 87":bool, "Boolean 88":bool, "Boolean 89":bool, "Boolean 90":bool, "Boolean 91":bool, "Boolean 92":bool, "Boolean 93":bool, "Boolean 94":bool, "Boolean 95":bool, "Boolean 96":bool, "Boolean 97":bool, "Boolean 98":bool, "Boolean 99":bool, "Boolean 100":bool}[], "ReTrain":bool, "TargDist":dbl[], "State":enum16{"Initialize", "Acquire Start", "Acquire Response", "Finalize"}, "KalmanType":enum16{"Standard", "Mean", "Refit", "LinSVReg", "NonLinSVReg", "PCA", "DWPRR", "AdaptKF", "NN", "NN_python", "AdaptKF2", "KF_Short_Goal"}, "EventStr":string, "SelElect":dbl, "KinSrc":enum16{"Off", "Training", "Decode", "COB", "LEAP"}, "HoverElect":dbl, "RasterWin":dbl, "WfCnt":dbl, "ClearWfs":bool, "ApplyThresh":bool, "ThreshVal":dbl, "ThreshMode":enum16{"RMS Single", "RMS All", "RMS Auto", "Volt Single", "Volt All"}, "DataFolder":string, "ClearEMG":bool, "KEMGClust":cluster{"Boolean 92":bool, "Boolean 82":bool, "Boolean 72":bool, "Boolean 62":bool, "Boolean 52":bool, "Boolean 42":bool, "Boolean 32":bool, "Boolean 22":bool, "Boolean 12":bool, "Boolean 2":bool, "Boolean 93":bool, "Boolean 83":bool, "Boolean 73":bool, "Boolean 63":bool, "Boolean 53":bool, "Boolean 43":bool, "Boolean 33":bool, "Boolean 23":bool, "Boolean 13":bool, "Boolean 3":bool, "Boolean 94":bool, "Boolean 84":bool, "Boolean 74":bool, "Boolean 64":bool, "Boolean 54":bool, "Boolean 44":bool, "Boolean 34":bool, "Boolean 24":bool, "Boolean 14":bool, "Boolean 4":bool, "Boolean 95":bool, "Boolean 85":bool, "Boolean 75":bool, "Boolean 65":bool, "Boolean 55":bool, "Boolean 45":bool, "Boolean 35":bool, "Boolean 25":bool, "Boolean 15":bool, "Boolean 5":bool, "Boolean 96":bool, "Boolean 86":bool, "Boolean 76":bool, "Boolean 66":bool, "Boolean 56":bool, "Boolean 46":bool, "Boolean 36":bool, "Boolean 26":bool, "Boolean 16":bool, "Boolean 6":bool, "Boolean 97":bool, "Boolean 87":bool, "Boolean 77":bool, "Boolean 67":bool, "Boolean 57":bool, "Boolean 47":bool, "Boolean 37":bool, "Boolean 27":bool, "Boolean 17":bool, "Boolean 7":bool, "Boolean 98":bool, "Boolean 88":bool, "Boolean 78":bool, "Boolean 68":bool, "Boolean 58":bool, "Boolean 48":bool, "Boolean 38":bool, "Boolean 28":bool, "Boolean 18":bool, "Boolean 8":bool, "Boolean 99":bool, "Boolean 89":bool, "Boolean 79":bool, "Boolean 69":bool, "Boolean 59":bool, "Boolean 49":bool, "Boolean 39":bool, "Boolean 29":bool, "Boolean 19":bool, "Boolean 9":bool}, "EvntFlag":bool, "FillUEA":bool, "FillEMG":bool, "FillMvnts":bool, "BadUEAElects":dbl[], "KEMGExtra":dbl[], "AllPairs":bool, "AutoThresh":dbl, "BadEMGChans":dbl[], "LinkedDOF":string, "AutoPopType":enum16{"Standard", "Stepwise", "Gram"}, "CARType":enum16{"Standard", "NN"}, "*Map":enum16{"pNeural/pEMG", "pNeural/aEMG", "aNeural/pEMG", "aNeural/aEMG"}, "GainFill":dbl, "ThreshFill":dbl, "TestType":enum16{"MSMS", "Bakeoff11", "Bakeoff21", "Bakeoff31", "Bakeoff32", "Bakeoff32_Ball", "Bakeoff32_Checkers", "Bakeoff32_Pen", "FragileBlock"}, "Outcome":enum16{"---", "Success", "Failure"}, "TrialCnt":dbl[][], "ClearTrials":bool, "Log10":bool, "KDFFile":string, "LimitExt":bool, "*Prosthesis":enum16{"MaleRight", "MaleLeft"}, "StartML":bool, "StartMLAux":bool, "StartRec":bool, "DynaThr":bool, "ModeFill":enum16{"Position", "Latching", "Leaky", "Velocity"}, "SpdFill":dbl, "DEKAMode":enum16{"Velocity", "Position"}, "FreeParam":dbl, "GoalNoise":dbl, "Load NN":bool, "ExportTrain":bool, "NumComp":enum16{"1 Computer", "2 Computers"}, "DataDir":string, "BuildDir":string, "LatchingFilter":bool, "Trigger":bool}
  T6 = typedef "FeedbackDecode_MvntClust.ctl" = cluster{"MvntType":cluster{"Thumb":enum8{"False", "True", "Mixed"}, "Index":enum8{"False", "True", "Mixed"}, "Middle":enum8{"False", "True", "Mixed"}, "Ring":enum8{"False", "True", "Mixed"}, "Little":enum8{"False", "True", "Mixed"}, "ThumbInt":enum8{"False", "True", "Mixed"}, "IndexInt":enum8{"False", "True", "Mixed"}, "RingInt":enum8{"False", "True", "Mixed"}, "LittleInt":enum8{"False", "True", "Mixed"}, "WristPitch":enum8{"False", "True", "Mixed"}, "WristYaw":enum8{"False", "True", "Mixed"}, "WristRoll":enum8{"False", "True", "Mixed"}}, "MvntParams":cluster{"Amp":dbl, "Delay":dbl, "Rise":dbl, "Hold":dbl}, "MvntList":cluster{"MvntMat":dbl[][], "MvntName":string, "Tracking":enum8{"False", "True", "Mixed"}, "Radius":dbl}[], "Set":bool, "Clear":bool, "Load":bool, "Mode":enum16{"Selected", "Block", "Random"}, "NTrials":dbl, "TargParams":cluster{"Gain":dbl, "Radius":dbl, "Acc":dbl}, "Save":bool, "PercTrials":dbl}
  T7 = cluster{"Thumb":dbl, "Index":dbl, "Middle":dbl, "Ring":dbl, "Little":dbl, "ThumbInt":dbl, "IndexInt":dbl, "RingInt":dbl, "LittleInt":dbl, "WristPitch":dbl, "WristYaw":dbl, "WristRoll":dbl}
  T8 = cluster{"Thumb":enum8{"False", "True", "Mixed"}, "Index":enum8{"False", "True", "Mixed"}, "Middle":enum8{"False", "True", "Mixed"}, "Ring":enum8{"False", "True", "Mixed"}, "Little":enum8{"False", "True", "Mixed"}, "ThumbInt":enum8{"False", "True", "Mixed"}, "IndexInt":enum8{"False", "True", "Mixed"}, "RingInt":enum8{"False", "True", "Mixed"}, "LittleInt":enum8{"False", "True", "Mixed"}, "WristPitch":enum8{"False", "True", "Mixed"}, "WristYaw":enum8{"False", "True", "Mixed"}, "WristRoll":enum8{"False", "True", "Mixed"}}
  T9 = typedef "FeedbackDecode_EncodeClust.ctl" = cluster{"ParamsTable":string[][], "Sel":bool[], "Stim":bool, "StimMode":enum16{"Off", "Manual", "MSMS", "VRE", "3DHand", "DEKA", "Analog(DEKA)"}, "StimStep":enum16{"Off", "1uA", "2uA", "5uA", "10uA", "20uA", "30uA"}[], "Jitter":bool, "Pulse":bool, "BFreq":dbl, "BAmp":dbl, "UEAArray":cluster{"Boolean 1":bool, "Boolean 2":bool, "Boolean 3":bool, "Boolean 4":bool, "Boolean 5":bool, "Boolean 6":bool, "Boolean 7":bool, "Boolean 8":bool, "Boolean 9":bool, "Boolean 10":bool, "Boolean 11":bool, "Boolean 12":bool, "Boolean 13":bool, "Boolean 14":bool, "Boolean 15":bool, "Boolean 16":bool, "Boolean 17":bool, "Boolean 18":bool, "Boolean 19":bool, "Boolean 20":bool, "Boolean 21":bool, "Boolean 22":bool, "Boolean 23":bool, "Boolean 24":bool, "Boolean 25":bool, "Boolean 26":bool, "Boolean 27":bool, "Boolean 28":bool, "Boolean 29":bool, "Boolean 30":bool, "Boolean 31":bool, "Boolean 32":bool, "Boolean 33":bool, "Boolean 34":bool, "Boolean 35":bool, "Boolean 36":bool, "Boolean 37":bool, "Boolean 38":bool, "Boolean 39":bool, "Boolean 40":bool, "Boolean 41":bool, "Boolean 42":bool, "Boolean 43":bool, "Boolean 44":bool, "Boolean 45":bool, "Boolean 46":bool, "Boolean 47":bool, "Boolean 48":bool, "Boolean 49":bool, "Boolean 50":bool, "Boolean 51":bool, "Boolean 52":bool, "Boolean 53":bool, "Boolean 54":bool, "Boolean 55":bool, "Boolean 56":bool, "Boolean 57":bool, "Boolean 58":bool, "Boolean 59":bool, "Boolean 60":bool, "Boolean 61":bool, "Boolean 62":bool, "Boolean 63":bool, "Boolean 64":bool, "Boolean 65":bool, "Boolean 66":bool, "Boolean 67":bool, "Boolean 68":bool, "Boolean 69":bool, "Boolean 70":bool, "Boolean 71":bool, "Boolean 72":bool, "Boolean 73":bool, "Boolean 74":bool, "Boolean 75":bool, "Boolean 76":bool, "Boolean 77":bool, "Boolean 78":bool, "Boolean 79":bool, "Boolean 80":bool, "Boolean 81":bool, "Boolean 82":bool, "Boolean 83":bool, "Boolean 84":bool, "Boolean 85":bool, "Boolean 86":bool, "Boolean 87":bool, "Boolean 88":bool, "Boolean 89":bool, "Boolean 90":bool, "Boolean 91":bool, "Boolean 92":bool, "Boolean 93":bool, "Boolean 94":bool, "Boolean 95":bool, "Boolean 96":bool, "Boolean 97":bool, "Boolean 98":bool, "Boolean 99":bool, "Boolean 100":bool}[], "AdjClust":cluster{"Add":bool, "Sub":bool, "Val":dbl[], "B":bool[], "Inc+":string[], "Set":bool, "LoadTable":bool, "SaveTable":bool, "ClearTable":bool, "DeleteSel":bool, "Inc-":string[]}, "PresetTable":string[][], "SelPreset":bool[], "SortClust":cluster{"Region":bool, "Receptor":bool, "Electrode":bool, "Min Amp":bool, "Max Amp":bool, "Min Freq":bool, "Max Freq":bool, "Duration":bool}, "SelSort":cluster{"Sel":bool}, "PresetClust":cluster{"Load":bool, "Clear":bool, "Save":bool, "Del":bool}, "RespClust":cluster{"RespType":enum16{"Sensor Map", "Full Map"}, "OpenResp":bool}, "AmpLimit":dbl, "FreqLimit":dbl, "DurLimit":dbl, "Wait Period":dbl, "Train Period":dbl}
  T10 = typedef "IMAQ Image.ctl" = refnum<image>
  T11 = cluster{"PupilConf":dbl, "PupilDia":dbl, "MdlConf":dbl, "PupilTS":dbl}
